vi "Configure Command.vi"(8 "Error In":errorcluster, 10 "Settings":T1 {"Linkages"."Linked Channel refnum" format="%.0x"}, 11 "C Refnum In":T2=18446744073709551615 format="%.0x") -> (0 "Error Out":errorcluster, 2 "Command Refnum":T2=18446744073709551615 format="%.0x", 3 "Message Refnum Out":T2=18446744073709551615 format="%.0x")   [LabVIEW 2020, in "Scripting API.lvlib"]
uses:
  Scripting API.lvlib
  <vilib>/NI VeriStand/Custom Device API/Custom Device Item Ref.ctl
  Examples/Control 5.ctl
  Examples/Control 15.ctl
  <vilib>/NI VeriStand/Custom Device API/Custom Device API.lvlib
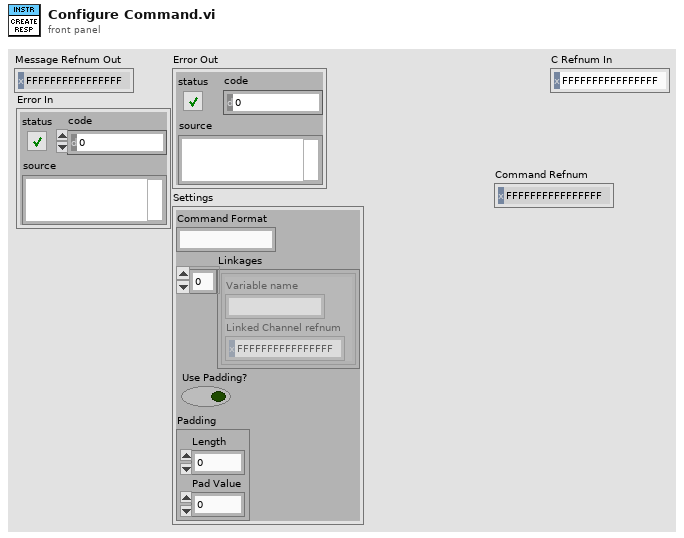
[diagram p1: front panel]
types:
  T1 = typedef "Control 5.ctl" = cluster{"Command Format":string, "Linkages":cluster{"Variable name":string, "Linked Channel refnum":T2}[], "Use Padding?":bool, "Padding":T3}
  T2 = typedef "Custom Device API.lvlib/Custom Device Item Ref.ctl" = u64
  T3 = typedef "Control 15.ctl" = cluster{"Length":u16, "Pad Value":u16}
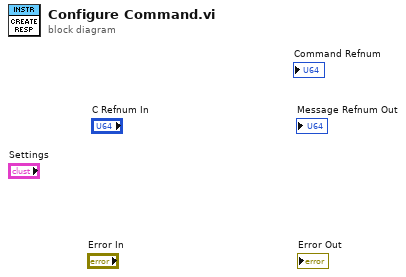
[diagram p0: block diagram]
diagram:
